vi "Intake Controller.vi"(8 "error in":errorcluster) -> ()   [LabVIEW 2019]
doc: "This VI executes continuously carrying out the current operation and responding to updates or new operations. It will often contain the timing or control code that is difficult to place directly in TeleOp. This VI generally opens all sensors and motors and isolates the rest of the robot code from knowing how the operations are carried out."
uses:
  <vilib>/Rock Robotics/WPI/Framework/Completion Status.ctl
  Intake Setpoints.ctl
  Intake Operations.ctl
  Intake Support Code/Pivot Position.ctl
  <vilib>/Rock Robotics/WPI/ThirdParty/REV Robotics/SPARK MAX/Typedef/Spark MAX Control Type.ctl
  <vilib>/Rock Robotics/Network Tables/NT Write Boolean.vi
panel:
  in  "Interactive Values":T1
  out "Current\nCmd":string
  in  "Buttons":cluster{"Execute Cmd":bool, "Abort Cmd":bool}
  out "Command Timing":cluster{"Start Time (ms)":u32, "Iterations":i32}
  out "Status":T4
  # "Tip: It may be helpful to observe inputs and sensor values.\nYou may also want to display tuning or debugging controls."
  # "Interactive Command: You may fill in the settings for a command\nand schedule it with the Execute button. You can observe and abort\nany command while fine tuning the code for the controller."
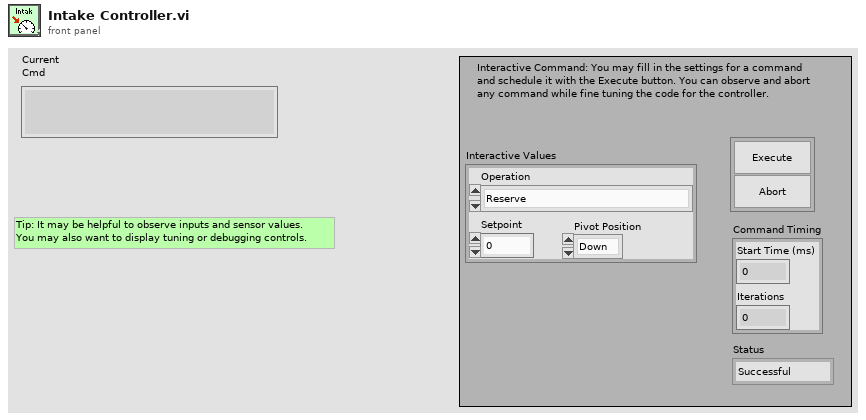
[diagram p1: front panel]
types:
  T1 = typedef "Intake Setpoints.ctl" = cluster{"Operation":T2, "Setpoint":dbl, "Pivot Position":T3}
  T2 = typedef "Intake Operations.ctl" = enum16{"Reserve", "Read Current", "Immediate", "Spin Rollers", "Pivot Position"}
  T3 = typedef "Pivot Position.ctl" = enum16{"Down", "Up"}
  T4 = typedef "Completion Status.ctl" = enum16{"Successful", "Aborted", "Incomplete"}
  T5 = cluster{"P Gain":dbl, "I Gain":dbl, "D Gain":dbl, "F Gain":dbl, "I Zone":dbl, "Min Output":dbl, "Max Output":dbl}
  T6 = typedef "WPI_MotorControlDeviceRef.ctl" = cluster{"DeviceStatus":errorcluster, "Type":T7, "PWM":cluster{"PWM Channel":T8, "DeadBand":T9}, "CAN":cluster{"Device Number":u8, "SetOutput VI Ref":variant, "GetOutput VI Ref":variant, "Enable VI Ref":variant, "Disable VI Ref":variant, "Data":variant}, "Invert":bool, "DIO PWM":cluster{"PWM \"Enable\" Channel":T8, "DIOChannel":T10, "PWM Rate":dbl}}
  T7 = typedef "WPI_MotorControlType.ctl" = enum16{"PWM", "CAN", "DIO PWM"}
  T8 = typedef "FPGA_DIOPWMChannel.ctl" = enum8{"PWM 0", "PWM 1", "PWM 2", "PWM 3", "PWM 4", "PWM 5", "PWM 6", "PWM 7", "PWM 8", "PWM 9", "PWM MXP 0", "PWM MXP 1", "PWM MXP 2", "PWM MXP 3", "PWM MXP 4", "PWM MXP 5", "PWM MXP 6", "PWM MXP 7", "PWM MXP 8", "PWM MXP 9", "Invalid"}
  T9 = typedef "WPI_PWMDeadband.ctl" = cluster{"Name":string, "maxPositivePwm":i32, "minPositivePwm":i32, "centerPwm":i32, "maxNegativePwm":i32, "minNegativePwm":i32, "angularRange":u16}
  T10 = typedef "FPGA_DIOChannel.ctl" = enum8{"DIO 0", "DIO 1", "DIO 2", "DIO 3", "DIO 4", "DIO 5", "DIO 6", "DIO 7", "DIO 8", "DIO 9", "DIO MXP 0", "DIO MXP 1", "DIO MXP 2", "DIO MXP 3", "DIO MXP 4", "DIO MXP 5", "DIO MXP 6", "DIO MXP 7", "DIO MXP 8", "DIO MXP 9", "DIO MXP 10", "DIO MXP 11", "DIO MXP 12", "DIO MXP 13", "DIO MXP 14", "DIO MXP 15", "SPI Port CS1", "SPI Port CS2", "SPI Port CS3", "SPI Port MISO", "SPI Port MOSI", "Invalid"}
  T11 = typedef "Command Status Info.ctl" = cluster{"Name":string, "Status":T4, "notifier out":T12}
  T12 = typedef "Completion Notifier.ctl" = refnum<notifier>
  T13 = cluster{"Current Command":T1, "Command Timing":cluster{"Start Time (ms)":u32, "Iterations":i32}, "Command Arguments":cluster{"Command Info":T11, "Description":string, "Default Command":T1, "queue out":refnum<queue>, "Subsystem Name":string}}
  T14 = typedef "Spark MAX Control Type.ctl" = enum16{"Percent VBus", "Voltage", "Velocity", "Position", "Smart Motion", "Current", "Smart Velocity"}
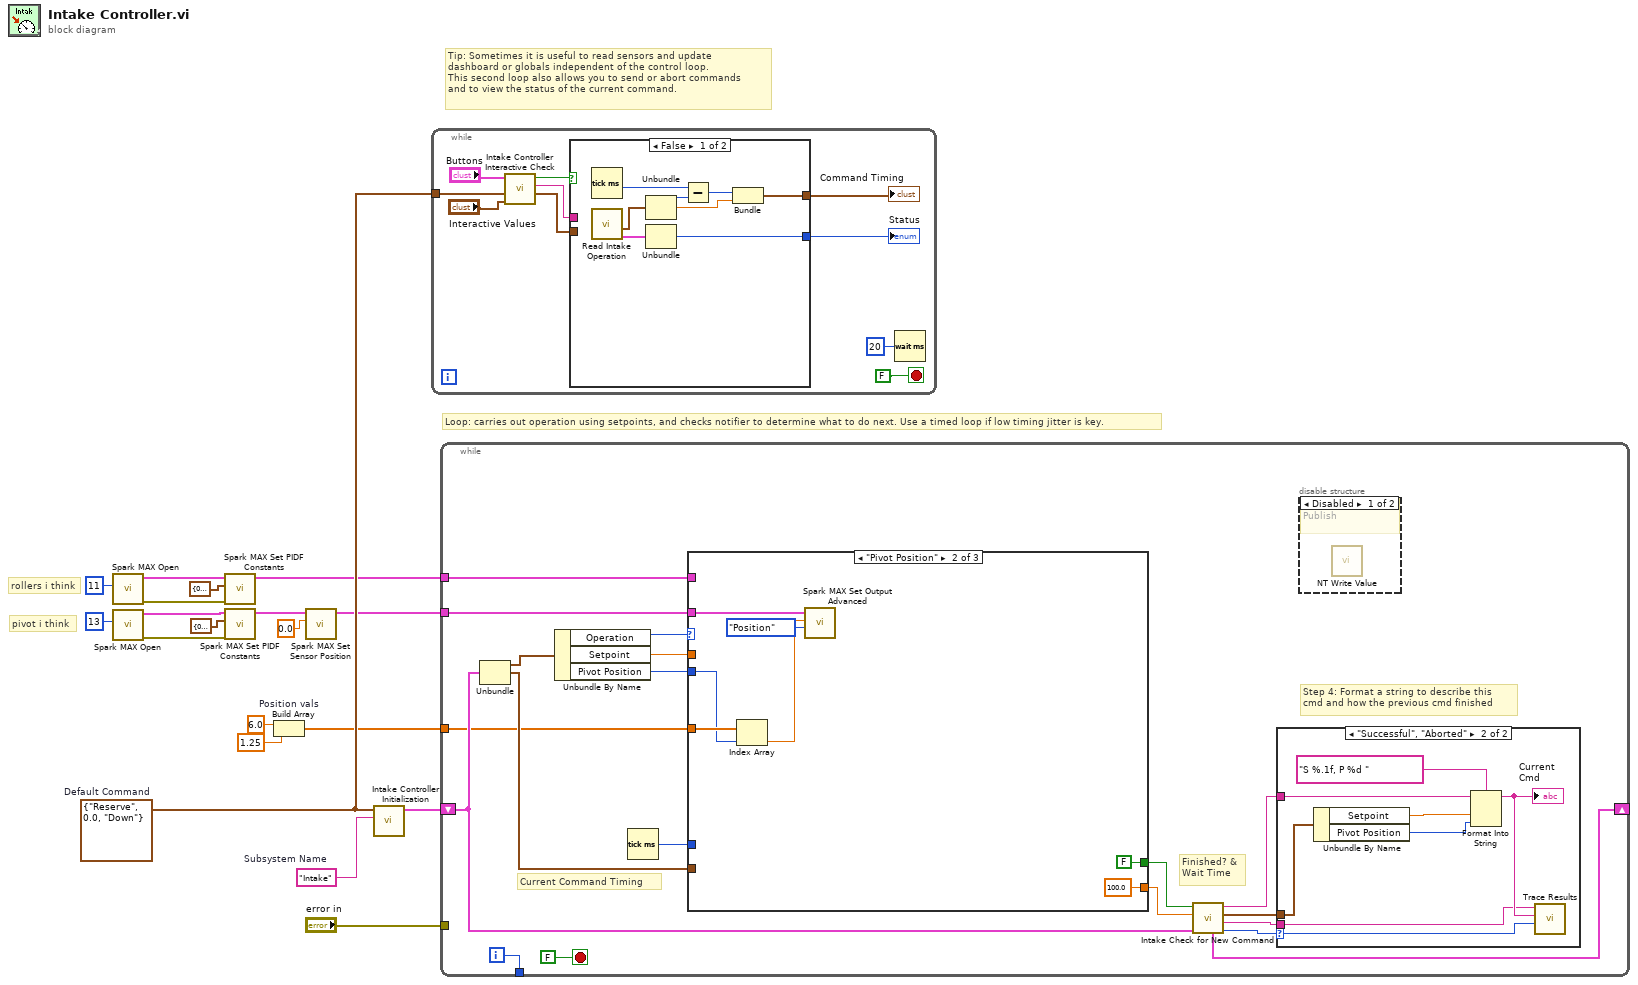
[diagram p0: block diagram]
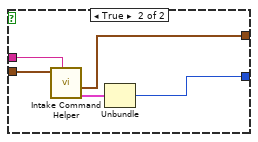
[diagram p2: hidden frame]
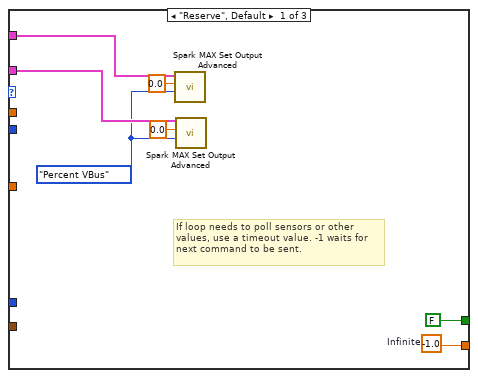
[diagram p5: hidden frame]
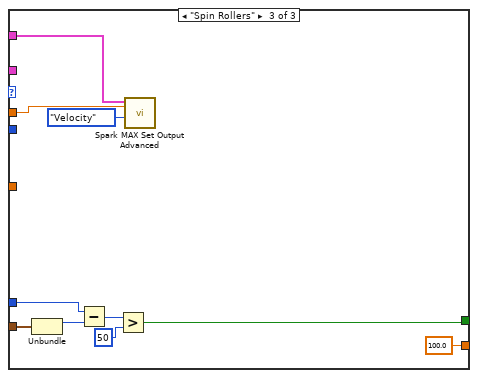
[diagram p6: hidden frame]
diagram:
  w16 = T1 {"Operation"=enum."Reserve", "Setpoint"=0.0, "Pivot Position"=enum."Down"}  # Default Command
  w17 = "Intake"  # Subsystem Name
  # "pivot i think"
  # "rollers i think"
  # "Tip: Sometimes it is useful to read sensors and update\ndashboard or globals independent of the control loop.\nThis second loop also allows you to send or abort commands\nand to view the status of the current command."
  # "Loop: carries out operation using setpoints, and checks notifier to determine what to do next. Use a timed loop if low timing jitter is key."
  n1 = call <vilib>:"Spark MAX Open.vi"("Device Number"=u8 11) -> ("error out"=w6:errorcluster, "MotorControlDeviceRef"=w9:T6)  [unwired: 9 in]
  n2 = call <vilib>:"Spark MAX Open.vi"("Device Number"=u8 13) -> ("error out"=w7:errorcluster, "MotorControlDeviceRef"=w8:T6)  [unwired: 9 in]
  n3 = call <vilib>:"Spark MAX Set PIDF Constants.vi"("error in"=w6, "PID Constants"=T5 {"P Gain"=0.0003, "I Gain"=0.0, "D Gain"=0.0, "F Gain"=0.0002, "I Zone"=0.0, "Min Output"=-1.0, "Max Output"=1.0}, "MotorControlDeviceRef"=w9) -> ("MotorControlDeviceRef"=w4:T6)  [unwired: 7 in, 1 out]
  n4 = call <vilib>:"Spark MAX Set PIDF Constants.vi"("error in"=w7, "PID Constants"=T5 {"P Gain"=0.07, "I Gain"=0.0001, "D Gain"=0.0, "F Gain"=0.0, "I Zone"=1.0, "Min Output"=-0.5, "Max Output"=0.5}, "MotorControlDeviceRef"=w8) -> ("MotorControlDeviceRef"=w13:T6)  [unwired: 7 in, 1 out]
  n5 = Build Array "Position vals"(6.0 ("element"), 1.25 ("element")) -> (w1:dbl[])
  n6 = call <vilib>:"Spark MAX Set Sensor Position.vi"("Position"=0.0, "MotorControlDeviceRef"=w13) -> ("MotorControlDeviceRef"=w5:T6)  [unwired: 8 in, 1 out]
  n7 = call "Intake Controller Initialization.vi"("Subsystem Name"=w17, "Default Command"=w16) -> ("Current Command"=w18:T13)  [unwired: 9 in]
  n8 = while {
    tunnel: w16 -> [w26]
    stop <- FALSE stop-if-true
    n9 = call "Intake Controller Interactive Check.vi"("Interactive Command in"="Interactive Values", "Default Command"=w26, "Buttons"="Buttons") -> ("Interactive Command out"=w23:T1, "Trace String"=w24:string, "Schedule"=w25:bool)  [unwired: 6 in]
    n10 = case shown="False" w25 {
      tunnel: [w37 w42] -> w22
      tunnel: w23 -> [_ w40]
      tunnel: [w33 w38] -> w21
      tunnel: w24 -> [_ w41]
      frame False {
        n11 = Tick Count (ms)() -> (millisecond timer value=w32:u32)
        n12 = call "Read Intake Operation.vi"() -> ("Command Info"=w30:T11, "SubSystem Data"=w31:T1)  [unwired: 9 in, 1 out]
        n13 = Unbundle(w31) -> ("Operation"=w36:T2, "Setpoint"=w34:dbl)  [unwired: 1 out]
        n14 = Unbundle(w30) -> ("Status"=w37:T4)  [unwired: 2 out]
        n15 = Subtract(x=w32, y=w36) -> (x-y=w35:u32)
        n16 = Bundle(w35, "Setpoint"=w34) -> (w33:cluster{u32, "Setpoint":dbl})  [unwired: 1 in]
      }
      frame True {
        n17 = call "Intake Command Helper.vi"("Description"=w41, "SubSystem Data"=w40) -> ("Command Info Out"=w39:T11, "Command Timing"=w38:cluster{"Start Time (ms)":u32, "Iterations":i32})  [unwired: 7 in, 1 out]
        n18 = Unbundle(w39) -> ("Status"=w42:T4)  [unwired: 2 out]
      }
    }
    "Status" <- w22
    "Command Timing" <- w21
    n19 = Wait (ms)(milliseconds to wait=u32 20) -> ()  [unwired: 1 out]
  }
  n20 = while {
    shift-right: [w54] -> _
    shift-left: w18 -> [w47]
    tunnel: [w60] -> _
    tunnel: "error in" -> [_]
    tunnel: w5 -> [w46]
    tunnel: w4 -> [w45]
    tunnel: w1 -> [w43]
    i -> [w60]
    stop <- FALSE stop-if-true
    # "Step 4: Format a string to describe this\ncmd and how the previous cmd finished"
    # "Current Command Timing"
    # "Finished? &\nWait Time"
    n21 = Unbundle(w47) -> ("Current Command"=w59:T1, "Command Timing"=w56:cluster{"Start Time (ms)":u32, "Iterations":i32})  [unwired: 1 out]
    n22 = Unbundle By Name(w59) -> ("Operation"=w58:T2, "Setpoint"=w55:dbl, "Pivot Position"=w44:T3)
    n23 = Tick Count (ms)() -> (millisecond timer value=w57:u32)
    n24 = case shown="\"Pivot Position\"" w58 {
      tunnel: [w76 100.0 ("Infinite") 100.0 ("Infinite")] -> w52
      tunnel: [FALSE ("ignore previous (F)") FALSE ("ignore previous (F)") w84] -> w53
      tunnel: w56 -> [_ _ w89]
      tunnel: w57 -> [_ _ w87]
      tunnel: w55 -> [_ _ w91]
      tunnel: w46 -> [w73 w83 _]
      tunnel: w45 -> [w74 _ w93]
      tunnel: w44 -> [_ w81 _]
      tunnel: w43 -> [_ w82 _]
      frame "Reserve", Default {
        w70 = Spark_MAX_Control_Type."Percent VBus" ("Control Mode")
        w76 = -1.0  # Infinite
        # "If loop needs to poll sensors or other\nvalues, use a timeout value. -1 waits for\nnext command to be sent."
        n25 = call <vilib>:"Spark MAX Set Output Advanced.vi"("Control Mode"=w70, "Setpoint"=0.0, "MotorControlDevRef"=w74) -> ()  [unwired: 7 in, 2 out]
        n26 = call <vilib>:"Spark MAX Set Output Advanced.vi"("Control Mode"=w70, "Setpoint"=0.0, "MotorControlDevRef"=w73) -> ()  [unwired: 7 in, 2 out]
      }
      frame "Pivot Position" {
        n27 = Index Array(array=w82, index=w81) -> (element=w80:dbl)
        n28 = call <vilib>:"Spark MAX Set Output Advanced.vi"("Control Mode"=Spark_MAX_Control_Type."Position", "Setpoint"=w80, "MotorControlDevRef"=w83) -> ()  [unwired: 7 in, 2 out]
      }
      frame "Spin Rollers" {
        n29 = Unbundle(w89) -> ("Start Time (ms)"=w88:u32)  [unwired: 1 out]
        n30 = Subtract(x=w87, y=w88) -> (x-y=w86:u32)
        n31 = Greater?(x=w86, y=u32 50) -> (0:w84:bool)
        n32 = call <vilib>:"Spark MAX Set Output Advanced.vi"("Control Mode"=Spark_MAX_Control_Type."Velocity", "Setpoint"=w91, "MotorControlDevRef"=w93) -> ()  [unwired: 7 in, 2 out]
      }
    }
    n33 = call "Intake Check for New Command.vi"("Current Command"=w47, "Wait time (ms)"=w52, "Finished?"=w53) -> ("Completion"=w48:T4, "Subsystem Name"=w49:string, "Current Command"=w50:T1, "Initial Trace String"=w51:string, "NextCommand"=w54:T13)  [unwired: 4 in]
    n34 = case shown="\"Successful\", \"Aborted\"" w48 {
      selector: w48 -> [_ w69]
      tunnel: w51 -> [_ w65]
      tunnel: w50 -> [_ w66]
      tunnel: w49 -> [_ w63]
      frame "Incomplete", Default {
        # "Continuing current command"
      }
      frame "Successful", "Aborted" {
        # "Report and setup for next command"
        n35 = Unbundle By Name(w66) -> ("Setpoint"=w68:dbl, "Pivot Position"=w62:T3)
        n36 = Format Into String(format string="S %.1f, P %d ", initial string=w65, w68, w62) -> (resulting string=w64:string)  [unwired: 1 in, 1 out]
        "Current\nCmd" <- w64
        n37 = call <vilib>:"Trace Results.vi"("Status of previous command"=w69, "Description"=w64, "Subsystem"=w63) -> ()  [unwired: 9 in]
      }
    }
    n38 = disable-structure shown="Disabled" {
      frame Disabled {
        # "Publish"
        n39 = call-poly <vilib>:"NT Write Value.vi"() -> ()  [unwired: 11 in, 1 out]
      }
      frame Enabled {
      }
    }
  }
